vi "switch task.vi"(2 "DigitalInputDevRef 2":T1, 3 "DigitalInputDevRef":T1) -> (0 "Angle Reset Switch":bool, 1 "Ball Switch":bool)   [LabVIEW 2011]
uses:
  <vilib>/Rock Robotics/WPI/DigitalInput/WPI_DigitalInputDevRef.ctl
  <vilib>/Rock Robotics/SystemInterfaces/DIO/FPGA_DIOChannel.ctl
  <vilib>/Rock Robotics/SystemInterfaces/Typedef/FPGA_TypedefDigitalModule.ctl
  Robot Global Data.vi
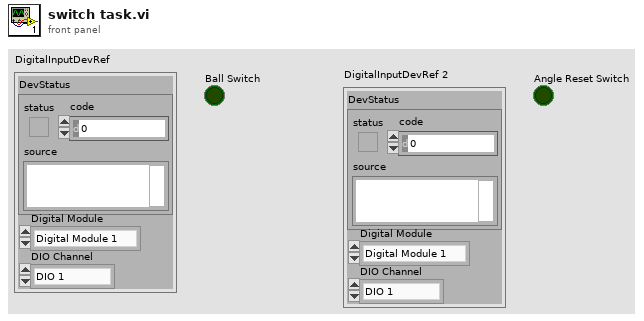
[diagram p1: front panel]
types:
  T1 = typedef "WPI_DigitalInputDevRef.ctl" = cluster{"DevStatus":errorcluster, "DIO Channel":T2, "Digital Module":T3}
  T2 = typedef "FPGA_DIOChannel.ctl" = enum8{"DIO 1", "DIO 2", "DIO 3", "DIO 4", "DIO 5", "DIO 6", "DIO 7", "DIO 8", "DIO 9", "DIO 10", "DIO 11", "DIO 12", "DIO 13", "DIO 14", "Invalid"}
  T3 = typedef "FPGA_TypedefDigitalModule.ctl" = enum16{"Digital Module 1", "Digital Module 2"}
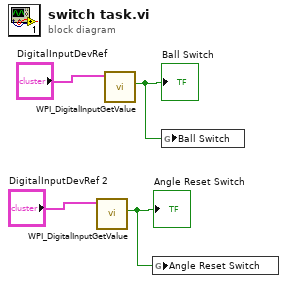
[diagram p0: block diagram]
diagram:
  n1 = call <vilib>:"WPI_DigitalInputGetValue.vi"("DigitalInputDevRef"="DigitalInputDevRef 2") -> ("Value"=w1:bool)  [unwired: 8 in, 2 out]
  "Angle Reset Switch" <- w1
  n2 = call <vilib>:"WPI_DigitalInputGetValue.vi"("DigitalInputDevRef"="DigitalInputDevRef") -> ("Value"=w3:bool)  [unwired: 8 in, 2 out]
  "Ball Switch" <- w3
  n3 = global write "Robot Global Data.vi" "Angle Reset Switch"(w1) -> ()
  n4 = global write "Robot Global Data.vi" "Ball Switch"(w3) -> ()
